vi "Write Cable Length.vi"(8 "error in (no error)":errorcluster, 10 "Cable Length (0: 0 m)":u32(ring)=1 items=["0 m", "1 m", "2 m", "3 m", "4 m"], 11 "Agilent 428x in":refnum<class "Agilent 428x.lvclass">) -> (0 "error out":errorcluster, 3 "Agilent 428x out":refnum<class "Agilent 428x.lvclass">)   [LabVIEW 2020, in "Agilent 428x.lvclass"]
uses:
  Agilent 428x.lvclass
  Agilent 428x.lvclass/Agilent 428x.ctl
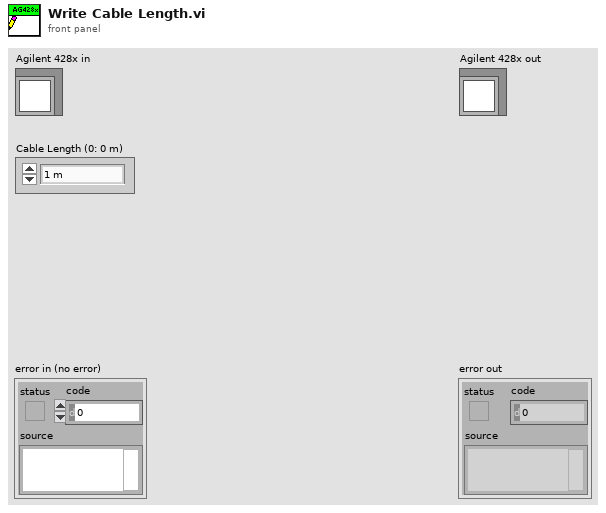
[diagram p1: front panel]
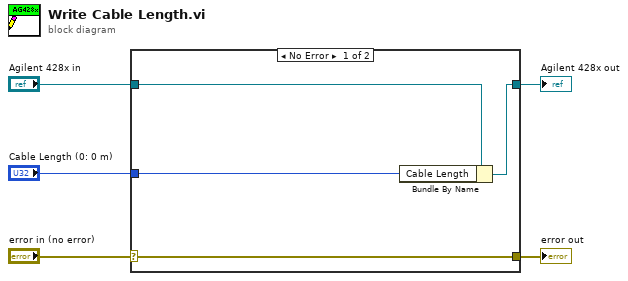
[diagram p0: block diagram]
diagram:
  n1 = case shown="No Error" "error in (no error)" {
    selector: "error in (no error)" -> [w9 w10]
    tunnel: [w9 w10] -> w4
    tunnel: [w7 w11] -> w2
    tunnel: "Agilent 428x in" -> [w8 w11]
    tunnel: "Cable Length (0: 0 m)" -> [w6 _]
    frame No Error {
      n2 = Bundle By Name(cluster=w8, "Cable Length"=w6) -> (w7:refnum<class "Agilent 428x.lvclass">)
    }
    frame Error {
    }
  }
  "error out" <- w4
  "Agilent 428x out" <- w2
